vi "injector magnet.vi"() -> ()   [LabVIEW 2016, in "features.lvlib"]
uses:
  Features/features/features.lvlib
  Features/features/field/Injector global.vi
  sub-VIs/sub-VIs.lvlib
panel:
  in  "reset injector":bool
  out "Property node error":errorcluster
  in  "oscillate":bool
  out "injector field":dbl
  in  "Stable 1 or 2":bool
  in  "Stable  Field  2":dbl
  in  "Scale":bool
  out "Stable or Rare 2":bool
  in  "Stable  Field":dbl
  in  "Rare Field":dbl(slide) scale=0.0..1.0
  in  "Stable or Rare":bool
  in  "stop":bool
  out "Waveform Chart":dbl(graph)
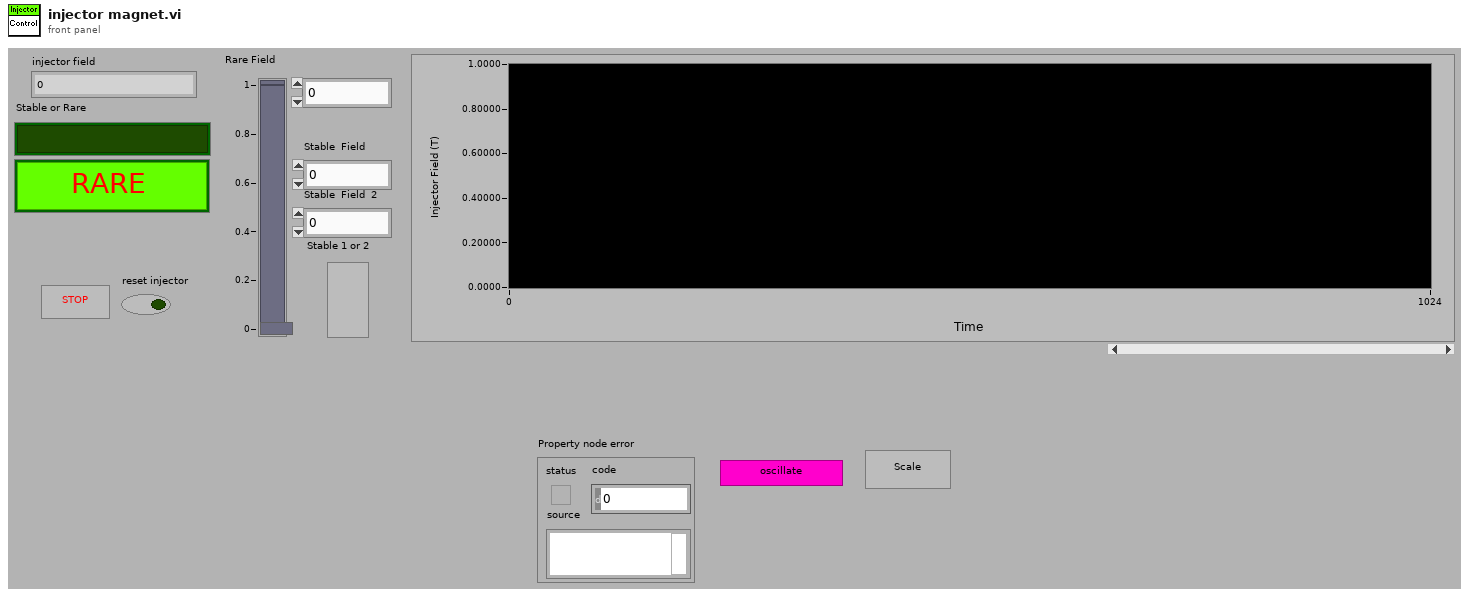
[diagram p1: front panel]
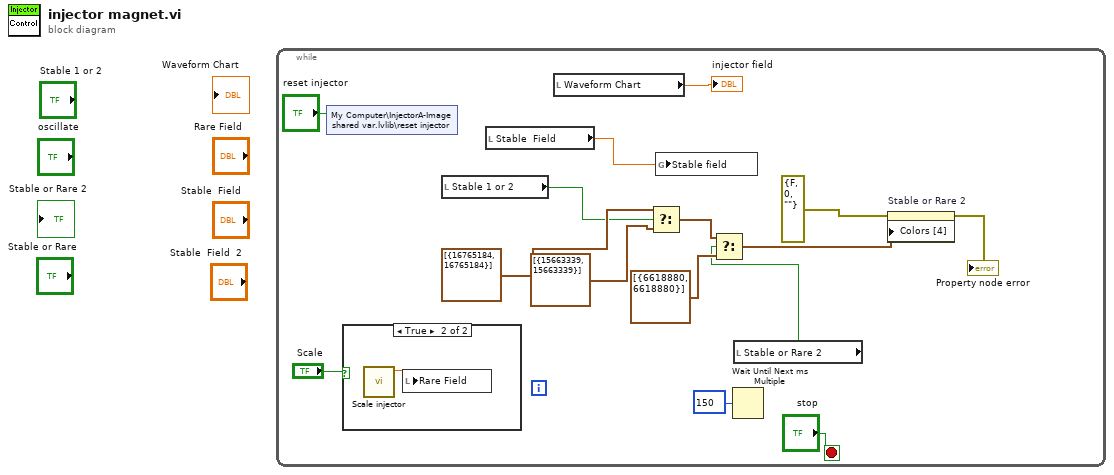
[diagram p0: block diagram]
diagram:
  n1 = while {
    stop <- "stop" stop-if-true
    n2 = shared-variable "My Computer\\InjectorA-Image shared var.lvlib\\reset injector"("reset injector") -> ()  [unwired: 1 in, 1 out]
    n3 = case shown="True" "Scale" {
      frame False {
      }
      frame True {
        n4 = call "Scale injector.vi"() -> ("Rare Field"=w16:dbl)  [unwired: 11 out]
        n5 = local write "Rare Field"(w16) -> ()
      }
    }
    n6 = local read "Stable 1 or 2"() -> (w5:bool)
    n7 = local read "Stable  Field"() -> (w7:dbl)
    n8 = local read "Waveform Chart"() -> (→"injector field":dbl)
    n9 = Select(t=cluster{u32, u32}[] [{16765184, 16765184}] ("Colors [4]"), s=w5, f=cluster{u32, u32}[] [{15663339, 15663339}] ("Colors [4]")) -> (s? t:f=w10:cluster{u32, u32}[])
    n10 = global write "Injector global.vi" "Stable field"(w7) -> ()
    n11 = Wait Until Next ms Multiple(millisecond multiple=u32 150) -> ()  [unwired: 1 out]
    n12 = local read "Stable or Rare 2"() -> (w6:bool)
    n13 = Select(t=w10, s=w6, f=cluster{u32, u32}[] [{6618880, 6618880}] ("Colors [4]")) -> (s? t:f=w11:cluster{u32, u32}[])
    n14 = property on="Stable or Rare 2" class="Bool (strict)"(error in=errorcluster {"status"=FALSE, "code"=0, "source"=""} ("error in (no error)"), "Colors [4]"=w11) -> (error out=→"Property node error":errorcluster)  [unwired: 1 in, 1 out]
  }
